vi "Generate PatchFolders.vi"(9 "Channel":enum16{"Green", "Red"}(ring)=enum."Red", 11 "ExperimentPath":path=path "D:/Srinivas/13 Patch Video/150610_14_10_33") -> (2 "Patch Image Folders":path[](array[path]))   [LabVIEW 2020]
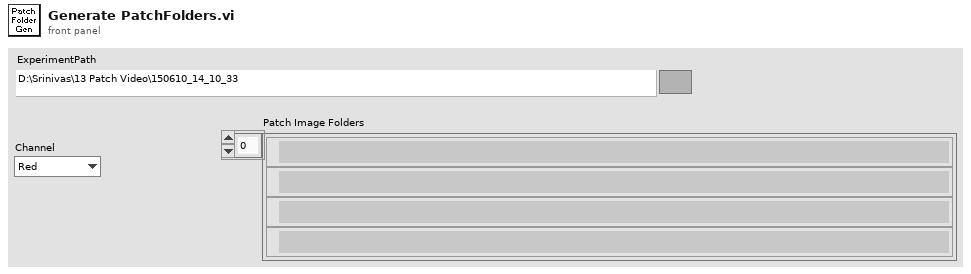
[diagram p1: front panel]
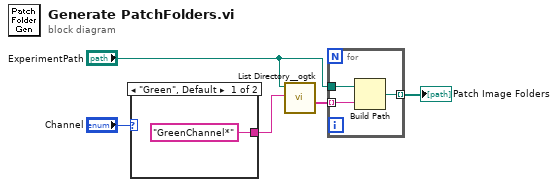
[diagram p0: block diagram]
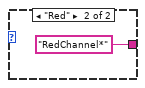
[diagram p2: hidden frame]
diagram:
  n1 = case shown="\"Green\", Default" "Channel" {
    tunnel: ["GreenChannel*" "RedChannel*"] -> w1
    frame "Green", Default {
    }
    frame "Red" {
    }
  }
  n2 = call <userlib>:"List Directory__ogtk.vi"("pattern"=w1, "directory path"="ExperimentPath") -> ("directory names"=w5:string[])  [unwired: 2 in, 3 out]
  n3 = for {
    tunnel: w5 -> [w10] mode=indexing
    tunnel: "ExperimentPath" -> [w9]
    tunnel: [w8] -> w3 mode=indexing
    n4 = Build Path(base path=w9, name or relative path=w10) -> (appended path=w8:path)
  }
  "Patch Image Folders" <- w3
